vi "PH_Stepmotor_BaseClass.update Axes PSDB Infos GUI.vi"(0 "VI in":refnum<vi>, 5 "error in (no error)":errorcluster) -> (14 "VI out":refnum<vi>, 19 "error out":errorcluster)   [LabVIEW 2014, in "PH_Stepmotor_BaseClass.lvlib"]
doc: "This VI is forseen to set Attributes to the related GUI element."
uses:
  PH_Stepmotor_BaseClass.lvlib
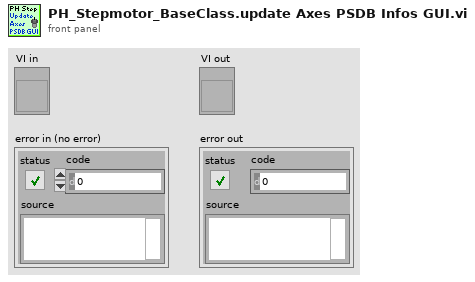
[diagram p1: front panel]
types:
  T1 = typedef "PH_Stepmotor_BaseClass.lvlib/PH_Stepmotor_BaseClass.i attribute.ctl" = cluster{"Device Error":errorcluster, "Axes PSDB Thread":cluster{"Ref":refnum<vi>, "Q-Ref":refnum<queue>, "Data Status":T2}, "Axes":T3[], "Axes PSDB Infos":cluster{"GUI Name":string, "PSDB Instance ID":i32, "PSDB Status Service ID":i32, "Axis":i32, "Class":string}[], "GUI Refs":T8}
  T2 = typedef "PH_PSDBWriter.lvlib/PH_PSDBWriter.Data Status.ctl" = i16
  T3 = typedef "PH_Stepmotor_BaseClass.lvlib/PH_Stepmotor_BaseClass.Axis Attributes.ctl" = cluster{"Settings":T4, "Endswitch?":bool, "DIM Service IDs":T6, "Activity":T7, "Configured?":bool, "Position":cluster{"Current":i32, "Target":i32}, "Position to set":cluster{"New?":bool, "Wanted":i32}, "Stop?":bool, "Reset?":bool, "Move?":bool, "Nothing connected?":bool}
  T4 = typedef "PH_Stepmotor_BaseClass.lvlib/PH_Stepmotor_BaseClass.Axis Settings.ctl" = cluster{"Sign change":bool, "Width":dbl, "Calibration":dbl, "Unit":string, "Motor Type":T5, "Unit Width":string, "Unit CF":string}
  T5 = typedef "PH_Stepmotor_BaseClass.lvlib/PH_Stepmotor_BaseClass.Motor Type.ctl" = enum16{"Unspecific", "OWIS 49.120.2633", "OWIS 49.060.1033", "OWIS 43.040.2558", "Diamond Motion 2200 series", "OWIS 49.120.266B.MV6", "Calorimeter", "Linear Stage 1", "MICOS VT-80", "MICOS VT-80 S", "Standa Rotstage nt0.95A", "PUF RA 320.200", "PUF RA 800.200", "PUF RA 800.400", "PUF RA 400.50", "1324.nn.800.50", "1324.n9c.800.50", "1324.nn.320.200", "1324.nn.400.200", "1324.nn.800.200", "1324.nn.400.50", "1324.8c9c.800.50", "1324.8c9c.400.200"}
  T6 = typedef "PH_Stepmotor_BaseClass.lvlib/PH_Stepmotor_BaseClass.Axis DIM Service IDs.ctl" = cluster{"Settings":i32, "Information":i32}
  T7 = typedef "PH_Stepmotor_BaseClass.lvlib/PH_Stepmotor_BaseClass.Axis Activity.ctl" = enum16{"No Information", "stopped", "running", "Failure", "Alarm", "stopped at backward ES", "stopped at foreward ES"}
  T8 = typedef "PH_Stepmotor_BaseClass.lvlib/PH_Stepmotor_BaseClass.GUI Refs.ctl" = cluster{"Axes Configuration":refnum<vi>, "Device Error":refnum<vi>, "Axes PSDB Infos":refnum<vi>}
  T9 = cluster{"GUI Name":string, "PSDB Instance ID":i32, "PSDB Status Service ID":i32, "Axis":i32, "Class":string}[]
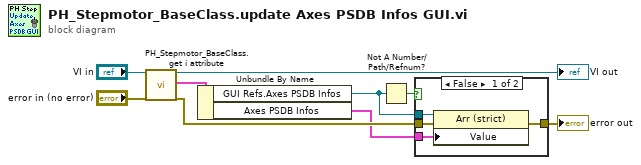
[diagram p0: block diagram]
diagram:
  n1 = call "PH_Stepmotor_BaseClass.get i attribute.vi"("i ref in"="VI in", "error in (no error)"="error in (no error)") -> ("i ref out"=→"VI out":refnum<vi>, "i attribute"=w4:T1, "error out"=w7:errorcluster)  [unwired: 15 in]
  n2 = Unbundle By Name(w4) -> ("GUI Refs.Axes PSDB Infos"=w2:refnum<vi>, "Axes PSDB Infos"=w1:T9)
  n3 = Not A Number/Path/Refnum?(number/path/refnum=w2) -> (NaN/Path/Refnum?=w3:bool)
  n4 = case shown="False" w3 {
    tunnel: w7 -> [w13 w14]
    tunnel: [w12 w14] -> w5
    tunnel: w2 -> [w11 _]
    tunnel: w1 -> [w10 _]
    frame False {
      n5 = property class="Arr (strict)"(reference=w11, error in=w13, "Value"=w10) -> (error out=w12:errorcluster)  [unwired: 1 out]
    }
    frame True {
    }
  }
  "error out" <- w5
